vi "外观 .vi"(0 "Data In":T5 caption="数据输入", 2 "Display State In":T2={"字符串长度"=0, "过滤字符"=[8, 127], "文本字体"={"Font Name"="", "Size"=0, "Bold"=FALSE, "Italic"=FALSE, "Underline"=FALSE, "Strikeout"=FALSE, "Color"=0}} caption="显示状态输入", 3 "Container State":T4 caption="容器状态") -> (6 "Data Out":T5 caption="数据输出", 7 "Display State Out":T2={"字符串长度"=0, "过滤字符"=[8, 127], "文本字体"={"Font Name"="", "Size"=0, "Bold"=FALSE, "Italic"=FALSE, "Underline"=FALSE, "Strikeout"=FALSE, "Color"=0}} caption="显示状态输出", 8 "Action":T1 caption="动作")   [LabVIEW 2013, in "Limit String.xctl"]
uses:
  Limit String.xctl
  <vilib>/_xctls/Container State.ctl
  <vilib>/Utility/miscctls.llb/LVFontTypeDef.ctl
  <vilib>/_xctls/Action.ctl
  <vilib>/_xctls/XControlSupport.lvlib
panel:
  in  "字符串":string
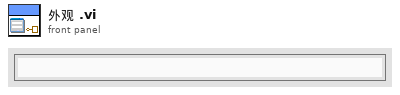
[diagram p1: front panel]
types:
  T1 = typedef "XControlSupport.lvlib/Action.ctl" = cluster{"Data Changed?":bool, "State Changed?":bool, "Action Name":string}
  T2 = typedef "Limit String.xctl/状态.ctl" = cluster{"字符串长度":u8, "过滤字符":i16[], "文本字体":T3}
  T3 = typedef "LVFontTypeDef.ctl" = cluster{"Font Name":string, "Size":u16, "Bold":bool, "Italic":bool, "Underline":bool, "Strikeout":bool, "Color":u32}
  T4 = typedef "XControlSupport.lvlib/Container State.ctl" = cluster{"Indicator?":bool, "Run Mode?":bool, " Refnum":refnum<vi>}
  T5 = typedef "Limit String.xctl/数据.ctl" = string
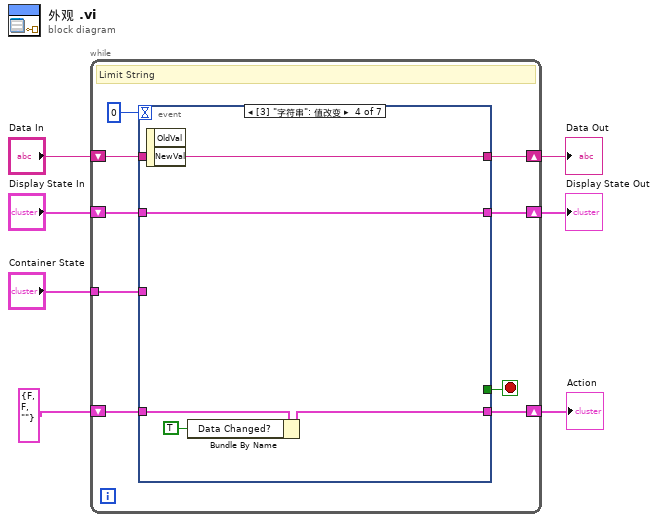
[diagram p0: block diagram]
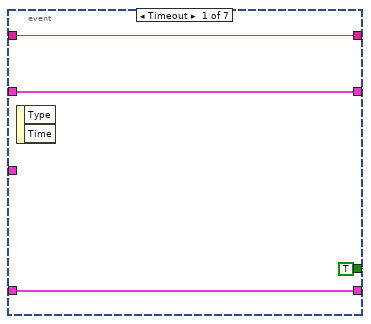
[diagram p2: hidden frame]
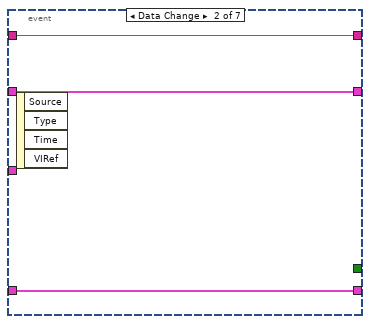
[diagram p3: hidden frame]
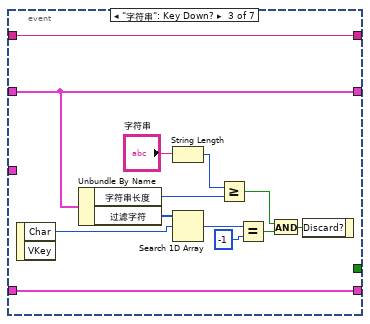
[diagram p4: hidden frame]
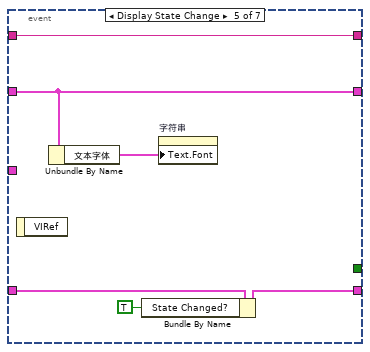
[diagram p5: hidden frame]
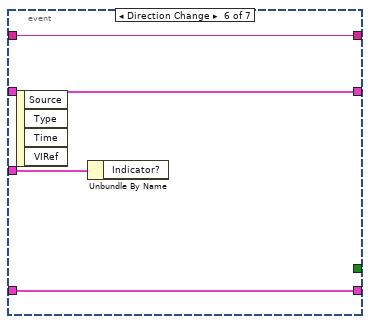
[diagram p6: hidden frame]
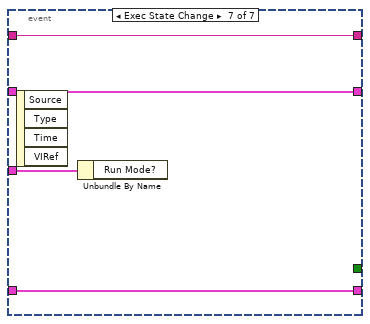
[diagram p7: hidden frame]
diagram:
  n1 = while {
    shift-right: [w15] -> w4
    shift-left: "Display State In" -> [w16]
    tunnel: "Container State" -> [w12]
    shift-right: [w10] -> w7
    shift-left: "Data In" -> [w11]
    shift-right: [w8] -> w2
    shift-left: T1 {"Data Changed?"=FALSE, "State Changed?"=FALSE, "Action Name"=""} ("Action") -> [w9]
    stop <- w14 stop-if-true
    # "Limit String"
    n2 = event shown="[3] \"字符串\": 值改变" {
      selector: _ -> [_ _ _ _ _ _ _]
      dyn-events: _ -> [_ _ _ _ _ _ _]
      timeout: 0 -> [_ _ _ _ _ _ _]
      tunnel: w16 -> [w18 w22 w34 w41 w45 w50 w53]
      tunnel: [w18 w22 w34 w41 w45 w50 w53] -> w15
      tunnel: [TRUE _ _ _ _ _ _] -> w14
      tunnel: w12 -> [_ _ _ _ _ w51 w55]
      tunnel: w11 -> [w17 w23 w24 _ w47 w49 w54]
      tunnel: [w17 w23 w24 w37 w47 w49 w54] -> w10
      tunnel: [w19 w21 w25 w39 w43 w48 w52] -> w8
      tunnel: w9 -> [w19 w21 w25 w40 w46 w48 w52]
      event Timeout {
        n3 = event-data() -> ()  [unwired: 1 in, 2 out]
      }
      event Data Change {
        n4 = event-data() -> ()  [unwired: 1 in, 4 out]
      }
      event "字符串": Key Down? {
        n5 = event-data() -> ("Char"=w32:i16)  [unwired: 1 in, 1 out]
        n6 = Unbundle By Name(w34) -> ("字符串长度"=w33:u8, "过滤字符"=w28:i16[])
        n7 = String Length(string="字符串") -> (length=w35:i32)
        n8 = Search 1D Array(1D array=w28, element=w32) -> (index of element=w31:i32)  [unwired: 1 in]
        n9 = Greater Or Equal?(x=w35, y=w33) -> (x >= y?=w36:bool)
        n10 = Equal?(x=w31, y=-1) -> (x = y?=w29:bool)
        n11 = And(x=w36, y=w29) -> (x .and. y?=w26:bool)
        n12 = event-data("Discard?"=w26) -> ()  [unwired: 1 in, 1 out]
      }
      event "字符串": Value Change {
        n13 = event-data() -> ("NewVal"=w37:string)  [unwired: 1 in, 1 out]
        n14 = Bundle By Name(cluster=w40, "Data Changed?"=TRUE) -> (w39:T1)
      }
      event Display State Change {
        n15 = event-data() -> ()  [unwired: 1 in, 1 out]
        n16 = Unbundle By Name(w45) -> ("文本字体"=w44:T3)
        n17 = Bundle By Name(cluster=w46, "State Changed?"=TRUE) -> (w43:T1)
        n18 = property on="字符串" class="Str"("Text.Font"=w44) -> ()  [unwired: 2 in, 2 out]
      }
      event Direction Change {
        n19 = event-data() -> ()  [unwired: 1 in, 4 out]
        n20 = Unbundle By Name(w51) -> ()  [unwired: 1 out]
      }
      event Exec State Change {
        n21 = event-data() -> ()  [unwired: 1 in, 4 out]
        n22 = Unbundle By Name(w55) -> ()  [unwired: 1 out]
      }
    }
  }
  "Display State Out" <- w4
  "Data Out" <- w7
  "Action" <- w2
